vi "encoder_logic.vi"(1 "encoder":fxp<+,4,4> format="%.0b") -> (0 "out":i16)   [LabVIEW 2019]
panel:
  # "A'B'AB"
  # "0\n1\n-1"
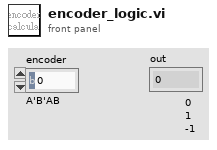
[diagram p1: front panel]
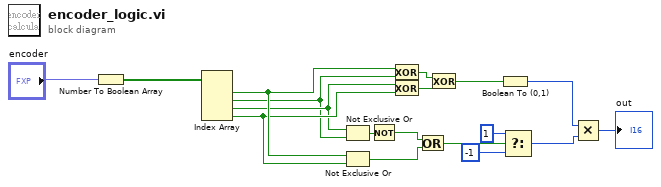
[diagram p0: block diagram]
diagram:
  n1 = Number To Boolean Array(number="encoder") -> (Boolean array=w15:bool[])
  n2 = Index Array(array=w15) -> (element #1=w14:bool, element #2=w11:bool, element #3=w12:bool, element #4=w13:bool)  [unwired: 4 in]
  n3 = Not Exclusive Or(1:w11, 2:w12) -> (0:w10:bool)
  n4 = Not Exclusive Or(1:w13, 2:w14) -> (0:w8:bool)
  n5 = Not(x=w10) -> (.not. x?=w9:bool)
  n6 = Exclusive Or(1:w11, 2:w14) -> (0:w16:bool)
  n7 = Exclusive Or(1:w13, 2:w12) -> (0:w17:bool)
  n8 = Or(x=w9, y=w8) -> (x .or. y?=w6:bool)
  n9 = Exclusive Or(1:w17, 2:w16) -> (0:w7:bool)
  n10 = Boolean To (0,1)(Boolean=w7) -> (0, 1=w3:i16)
  n11 = Select(t=i16 1, s=w6, f=i16 -1) -> (s? t:f=w2:i16)
  n12 = Multiply(x=w3, y=w2) -> (x*y=→"out":i16)
